vi "UPCODE.vi"(0 "CODE_SENSOR":string, 5 "CODE_MAIN":string, 11 "错误输入":errorcluster) -> (15 "error out":errorcluster)   [LabVIEW 2020]
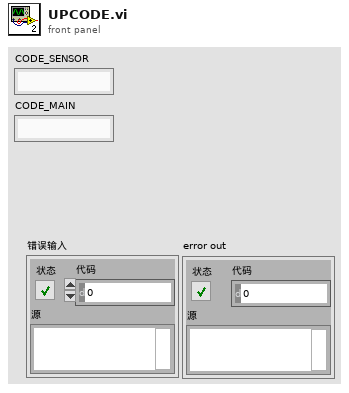
[diagram p1: front panel]
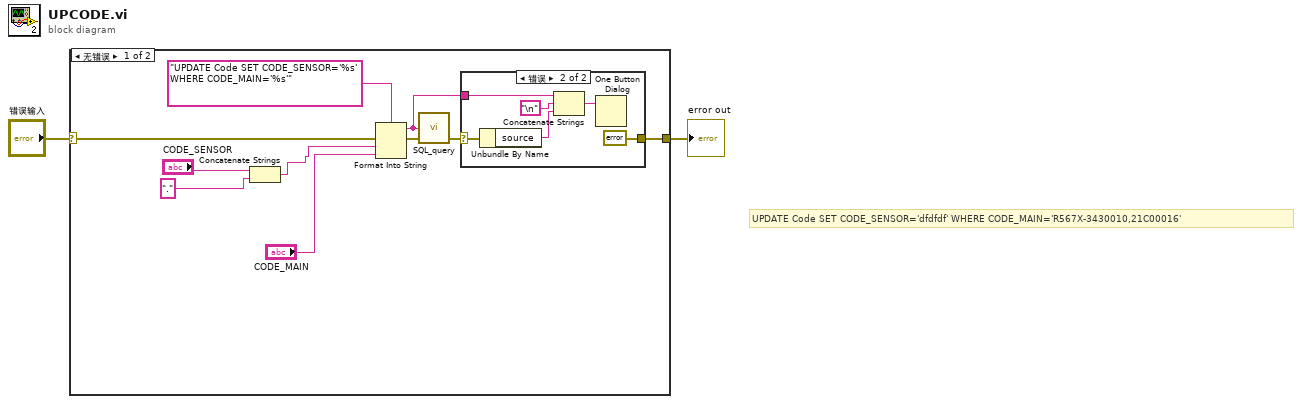
[diagram p0: block diagram]
diagram:
  # "UPDATE Code SET CODE_SENSOR='dfdfdf' WHERE CODE_MAIN='R567X-3430010,21C00016'"
  n1 = case shown="无错误" "错误输入" {
    selector: "错误输入" -> [w9 w20]
    tunnel: [w7 w20] -> w1
    frame No Error {
      n2 = Concatenate Strings("CODE_SENSOR", ".") -> (w3:string)
      n3 = Format Into String(format string="UPDATE Code SET CODE_SENSOR='%s' WHERE CODE_MAIN='%s'", error in=w9, w3, "CODE_MAIN") -> (resulting string=w6:string, error out=w12:errorcluster)  [unwired: 1 in]
      n4 = call "SQL_query.vi"("error in (no error)"=w12, "SQL query"=w6) -> ("error out"=w8:errorcluster)  [unwired: 2 in, 1 out]
      n5 = case shown="错误" w8 {
        selector: w8 -> [w13 w17]
        tunnel: [w13 errorcluster {"status"=FALSE, "code"=0, "source"=""} ("error IO")] -> w7
        tunnel: w6 -> [_ w19]
        frame No Error {
        }
        frame Error {
          n6 = Unbundle By Name(w17) -> ("source"=w16:string)
          n7 = Concatenate Strings(w19, "\n", w16) -> (w15:string)
          n8 = One Button Dialog(message=w15) -> ()  [unwired: 1 in, 1 out]
        }
      }
    }
    frame Error {
    }
  }
  "error out" <- w1
